vi "IBM4_Open.vi"(9 "Mode":enum16{"DC", "AC"}(ring), 11 "COM Port":refnum<visa-resource-name>) -> (0 "error out":errorcluster, 2 "UCC Revision #":string, 3 "COM resource out":refnum<visa-resource-name>)   [LabVIEW 2021, in "IBM4.lvlib"]
doc: "This VI is used to open the IBM4 (Itsybitsy M4). This should always be the first VI called, when communicating with the IBM4. \n\nThe COM Port must be the correct one for the IBM4, or else an error will be returned. In addition, if the IBM4 has not been loaded with the correct Circuit Python code, an error will also be generated.\n\nIf a properly configure IBM4 exists at that port, then the UCC Revision # will be returned.\n\nRemember to also close the device at the end. If this is not done, you may need to reboot your computer to free up resources."
uses:
  <instrlib>/IBM4/IBM4.lvlib
  <vilib>/Instr/_visa.llb/VISA Configure Serial Port (Instr).vi
panel:
  out "The Mode returned":string
  out "read buffer":string
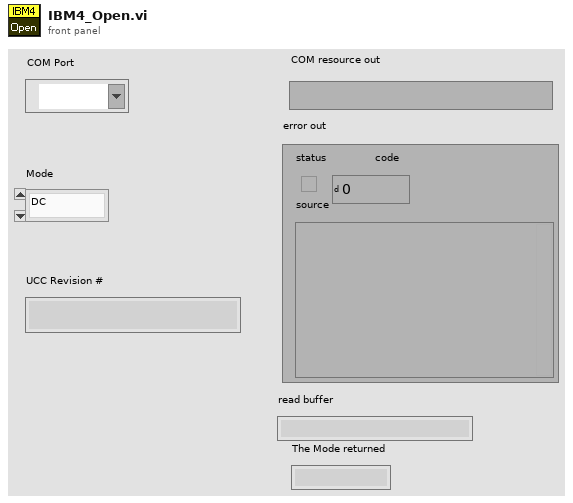
[diagram p1: front panel]
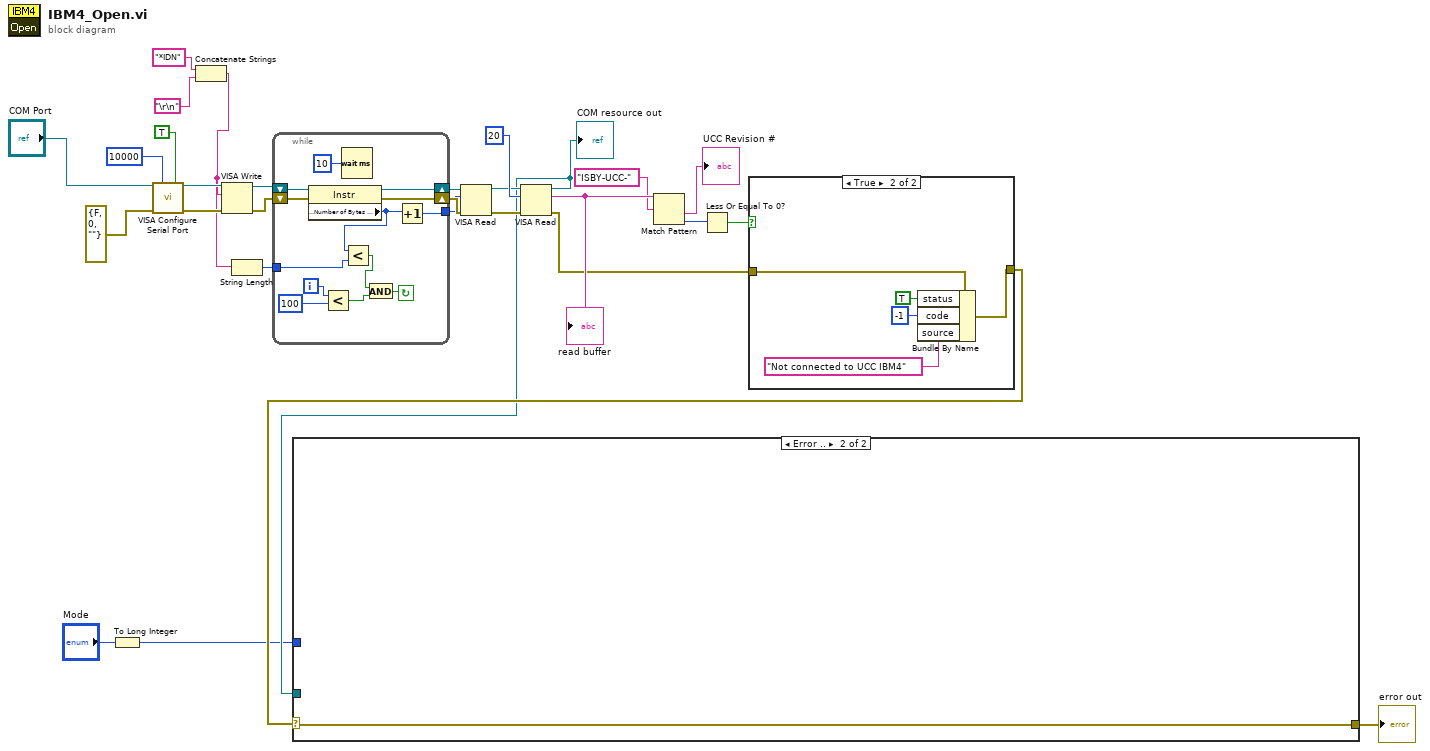
[diagram p0: block diagram]
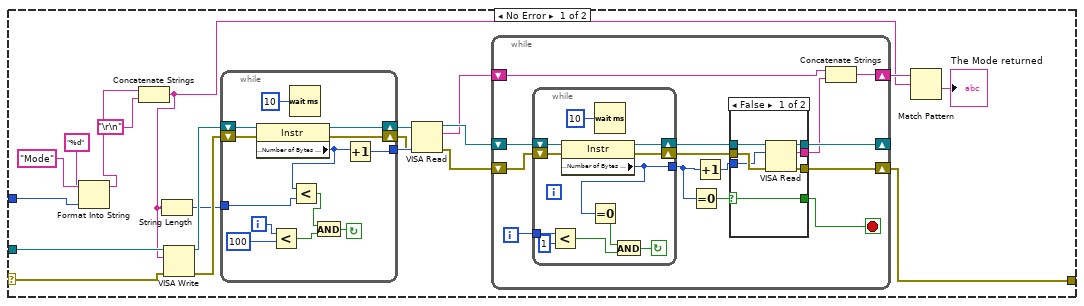
[diagram p2: hidden frame]
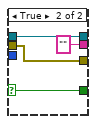
[diagram p3: hidden frame]
diagram:
  n1 = To Long Integer(number="Mode") -> (32bit integer=w1:i32)
  n2 = call-poly "VISA Configure Serial Port"("VISA resource name"="COM Port", "timeout (10sec)"=u32 10000, "Enable Termination\nChar (T)"=TRUE ("Enable Termination\nChar (T)"), "error in (no error)"=errorcluster {"status"=FALSE, "code"=0, "source"=""}) -> ("VISA resource name out"=w26:refnum<visa-resource-name>, "error out"=w25:errorcluster)  [unwired: 10 in]
  n3 = Concatenate Strings("*IDN" ("write buffer"), "\r\n") -> (w14:string)
  n4 = VISA Write(VISA resource name=w26, write buffer=w14, error in (no error)=w25) -> (VISA resource name out=w21:refnum<visa-resource-name>, error out=w20:errorcluster)  [unwired: 1 out]
  n5 = String Length(string=w14) -> (length=w13:i32)
  n6 = while {
    tunnel: [w31] -> w17
    shift-right: [w41] -> w19
    shift-left: w21 -> [w42]
    shift-right: [w39] -> w18
    shift-left: w20 -> [w40]
    tunnel: w13 -> [w37]
    i -> [w32]
    stop <- w35 continue-if-true
    n7 = property class="Instr"(reference=w42, error in=w40) -> (reference out=w41:refnum<visa-resource-name>, error out=w39:errorcluster, "Serial Settings:Number of Bytes at Serial Port"=w30:u32)
    n8 = Less?(x=w32, y=100) -> (x < y?=w34:bool)
    n9 = Wait (ms)(milliseconds to wait=u32 10) -> ()  [unwired: 1 out]
    n10 = Less?(x=w30, y=w37) -> (x < y?=w33:bool)
    n11 = And(x=w33, y=w34) -> (x .and. y?=w35:bool)
    n12 = Increment(x=w30) -> (x+1=w31:u32)
  }
  n13 = VISA Read(VISA resource name=w19, byte count=w17, error in (no error)=w18) -> (VISA resource name out=w16:refnum<visa-resource-name>, error out=w15:errorcluster)  [unwired: 2 out]
  n14 = VISA Read(VISA resource name=w16, byte count=u32 20, error in (no error)=w15) -> (VISA resource name out=w3:refnum<visa-resource-name>, read buffer=w12:string, error out=w8:errorcluster)  [unwired: 1 out]
  "COM resource out" <- w3
  "read buffer" <- w12
  n15 = Match Pattern(string=w12, regular expression="ISBY-UCC-" ("format string")) -> (after substring=→"UCC Revision #":string, offset past match=w9:i32)  [unwired: 1 in, 2 out]
  n16 = Less Or Equal To 0?(x=w9) -> (x <= 0?=w7:bool)
  n17 = case shown="True" w7 {
    tunnel: w8 -> [w43 w46]
    tunnel: [w43 w47] -> w5
    frame False {
    }
    frame True {
      n18 = Bundle By Name(cluster=w46, "status"=TRUE, "code"=-1, "source"="Not connected to UCC IBM4") -> (w47:errorcluster)
    }
  }
  n19 = case shown="Error .." w5 {
    selector: w5 -> [w67 w118]
    tunnel: [w49 w118] -> w4
    tunnel: w3 -> [w66 _]
    tunnel: w1 -> [w63 _]
    frame No Error {
      n20 = Format Into String(format string="%d", initial string="Mode" ("write buffer"), w63) -> (resulting string=w62:string)  [unwired: 1 in, 1 out]
      n21 = Concatenate Strings(w62, "\r\n") -> (w51:string)
      n22 = String Length(string=w51) -> (length=w56:i32)
      n23 = VISA Write(VISA resource name=w66, write buffer=w51, error in (no error)=w67) -> (VISA resource name out=w58:refnum<visa-resource-name>, error out=w57:errorcluster)  [unwired: 1 out]
      n24 = while {
        tunnel: [w106] -> w60
        shift-right: [w116] -> w61
        shift-left: w58 -> [w117]
        shift-right: [w114] -> w59
        shift-left: w57 -> [w115]
        tunnel: w56 -> [w112]
        i -> [w107]
        stop <- w110 continue-if-true
        n25 = property class="Instr"(reference=w117, error in=w115) -> (reference out=w116:refnum<visa-resource-name>, error out=w114:errorcluster, "Serial Settings:Number of Bytes at Serial Port"=w105:u32)
        n26 = Less?(x=w107, y=100) -> (x < y?=w109:bool)
        n27 = Wait (ms)(milliseconds to wait=u32 10) -> ()  [unwired: 1 out]
        n28 = Less?(x=w105, y=w112) -> (x < y?=w108:bool)
        n29 = And(x=w108, y=w109) -> (x .and. y?=w110:bool)
        n30 = Increment(x=w105) -> (x+1=w106:u32)
      }
      n31 = VISA Read(VISA resource name=w61, byte count=w60, error in (no error)=w59) -> (VISA resource name out=w55:refnum<visa-resource-name>, read buffer=w53:string, error out=w54:errorcluster)  [unwired: 1 out]
      n32 = while {
        shift-right: [w82] -> _
        shift-left: w55 -> [w80]
        shift-right: [w81] -> w49
        shift-left: w54 -> [w78]
        shift-right: [w76] -> w52
        shift-left: w53 -> [w74]
        i -> [w73]
        stop <- w69 stop-if-true
        n33 = while {
          tunnel: [w99] -> w72
          shift-right: [w103] -> w79
          shift-left: w80 -> [w104]
          shift-right: [w101] -> w77
          shift-left: w78 -> [w102]
          tunnel: w73 -> [w98]
          stop <- w96 continue-if-true
          n34 = Less?(x=w98, y=1) -> (x < y?=w95:bool)
          n35 = property class="Instr"(reference=w104, error in=w102) -> (reference out=w103:refnum<visa-resource-name>, error out=w101:errorcluster, "Serial Settings:Number of Bytes at Serial Port"=w99:u32)
          n36 = Equal To 0?(x=w99) -> (x = 0?=w94:bool)
          n37 = Wait (ms)(milliseconds to wait=u32 10) -> ()  [unwired: 1 out]
          n38 = And(x=w94, y=w95) -> (x .and. y?=w96:bool)
        }
        n39 = Equal To 0?(x=w72) -> (x = 0?=w70:bool)
        n40 = Increment(x=w72) -> (x+1=w71:u32)
        n41 = case shown="False" w70 {
          selector: w70 -> [w83 w92]
          tunnel: [w89 w93] -> w82
          tunnel: [w88 w91] -> w81
          tunnel: w79 -> [w87 w93]
          tunnel: w77 -> [w86 w91]
          tunnel: [w85 "" ("read buffer")] -> w75
          tunnel: w71 -> [w84 _]
          tunnel: [w83 w92] -> w69
          frame False {
            n42 = VISA Read(VISA resource name=w87, byte count=w84, error in (no error)=w86) -> (VISA resource name out=w89:refnum<visa-resource-name>, read buffer=w85:string, error out=w88:errorcluster)  [unwired: 1 out]
          }
          frame True {
          }
        }
        n43 = Concatenate Strings(w74, w75) -> (w76:string)
      }
      n44 = Match Pattern(string=w52, regular expression=w51) -> (after substring=→"The Mode returned":string)  [unwired: 1 in, 3 out]
    }
    frame Error {
    }
  }
  "error out" <- w4
